vi "Layout - JSON escape string.vi"() -> ()   [LabVIEW 2026, in "Tests.lvlib"]
uses:
  Tests.lvlib
  <vilib>/addons/_JKI Toolkits/Caraya/classes/Assert/Assert Equal Value_Variant.vi
  <vilib>/addons/_JKI Toolkits/Caraya/classes/Test/Test.lvclass
  src/Lumberjack.lvlib
  <vilib>/addons/_JKI Toolkits/Caraya/classes/Assert/Assert.lvclass
panel:
  out "error out":errorcluster
  in  "error in (no error)":errorcluster
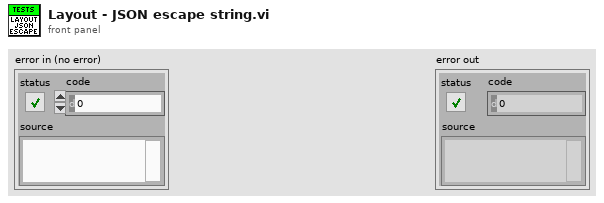
[diagram p1: front panel]
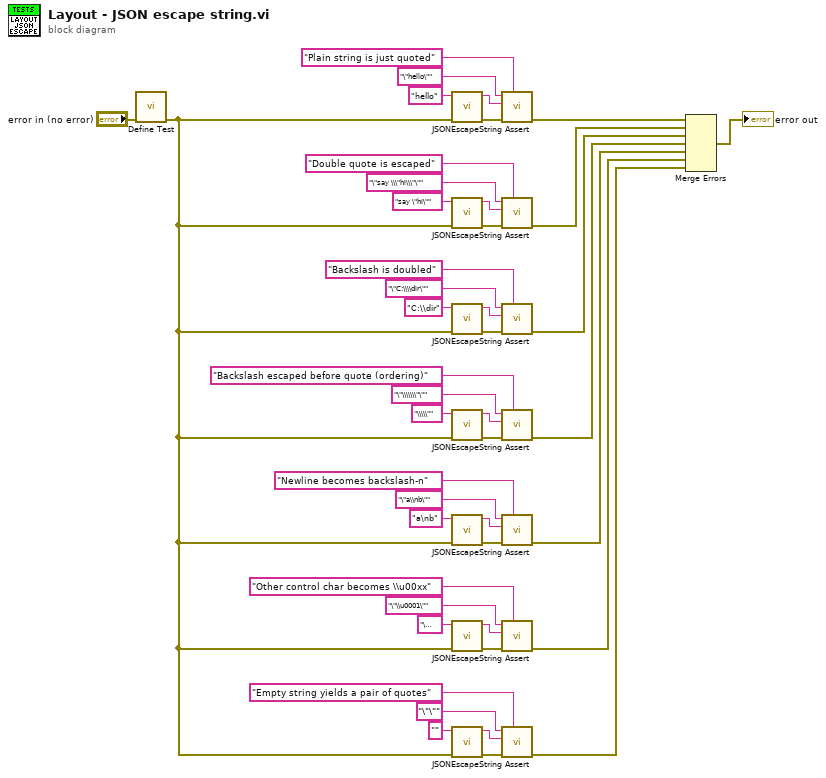
[diagram p0: block diagram]
diagram:
  n1 = call <vilib>:"Define Test.vi"("error in (no error)"="error in (no error)") -> ("error out"=w7:errorcluster)  [unwired: 9 in, 1 out]
  n2 = call "JSONEscapeString.vi"("error in (no error)"=w7, "raw"="hello") -> ("error out"=w43:errorcluster, "escaped"=w41:string)  [unwired: 8 in]
  n3 = call "JSONEscapeString.vi"("error in (no error)"=w7, "raw"="say \"hi\"") -> ("error out"=w37:errorcluster, "escaped"=w35:string)  [unwired: 8 in]
  n4 = call "JSONEscapeString.vi"("error in (no error)"=w7, "raw"="C:\\dir") -> ("error out"=w32:errorcluster, "escaped"=w30:string)  [unwired: 8 in]
  n5 = call "JSONEscapeString.vi"("error in (no error)"=w7, "raw"="\\\\\"") -> ("error out"=w27:errorcluster, "escaped"=w25:string)  [unwired: 8 in]
  n6 = call "JSONEscapeString.vi"("error in (no error)"=w7, "raw"="a\nb") -> ("error out"=w22:errorcluster, "escaped"=w20:string)  [unwired: 8 in]
  n7 = call "JSONEscapeString.vi"("error in (no error)"=w7, "raw"="\u0001") -> ("error out"=w17:errorcluster, "escaped"=w15:string)  [unwired: 8 in]
  n8 = call "JSONEscapeString.vi"("error in (no error)"=w7, "raw"="") -> ("error out"=w12:errorcluster, "escaped"=w10:string)  [unwired: 8 in]
  n9 = call-poly <vilib>:"Assert.vi"("Label"="Plain string is just quoted", "error in (no error)"=w43, "Actual"=w41, "Expected"="\"hello\"" ("raw")) -> ("error out"=w39:errorcluster)  [unwired: 6 in, 1 out]
  n10 = call-poly <vilib>:"Assert.vi"("Label"="Double quote is escaped", "error in (no error)"=w37, "Actual"=w35, "Expected"="\"say \\\"hi\\\"\"" ("raw")) -> ("error out"=w6:errorcluster)  [unwired: 6 in, 1 out]
  n11 = call-poly <vilib>:"Assert.vi"("Label"="Backslash is doubled", "error in (no error)"=w32, "Actual"=w30, "Expected"="\"C:\\\\dir\"" ("raw")) -> ("error out"=w5:errorcluster)  [unwired: 6 in, 1 out]
  n12 = call-poly <vilib>:"Assert.vi"("Label"="Backslash escaped before quote (ordering)", "error in (no error)"=w27, "Actual"=w25, "Expected"="\"\\\\\\\"\"" ("raw")) -> ("error out"=w4:errorcluster)  [unwired: 6 in, 1 out]
  n13 = call-poly <vilib>:"Assert.vi"("Label"="Newline becomes backslash-n", "error in (no error)"=w22, "Actual"=w20, "Expected"="\"a\\nb\"" ("raw")) -> ("error out"=w3:errorcluster)  [unwired: 6 in, 1 out]
  n14 = call-poly <vilib>:"Assert.vi"("Label"="Other control char becomes \\u00xx", "error in (no error)"=w17, "Actual"=w15, "Expected"="\"\\u0001\"" ("raw")) -> ("error out"=w2:errorcluster)  [unwired: 6 in, 1 out]
  n15 = call-poly <vilib>:"Assert.vi"("Label"="Empty string yields a pair of quotes", "error in (no error)"=w12, "Actual"=w10, "Expected"="\"\"" ("raw")) -> ("error out"=w1:errorcluster)  [unwired: 6 in, 1 out]
  n16 = Merge Errors(w39, w6, w5, w4, w3, w2, w1) -> (→"error out":errorcluster)
